vi "DHT12 Get Humidity.vi"(1 "Data":u8[](array[numeric])) -> (0 "Humidity":dbl)   [LabVIEW 2020, in "lv_dht12.lvlib"]
uses:
  lv_dht12.lvlib
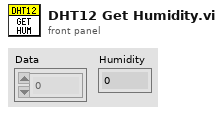
[diagram p1: front panel]
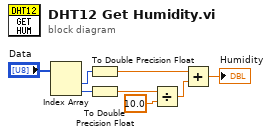
[diagram p0: block diagram]
diagram:
  n1 = Index Array(array="Data") -> (element #1=w5:u8, element #2=w4:u8)  [unwired: 2 in]
  n2 = To Double Precision Float(number=w5) -> (double precision float=w8:dbl)
  n3 = To Double Precision Float(number=w4) -> (double precision float=w7:dbl)
  n4 = Divide(x=w7, y=10.0) -> (x/y=w3:dbl)
  n5 = Add(x=w8, y=w3) -> (x+y=→"Humidity":dbl)
